vi "RT_Aerodynamic_Moment_due_to_Fins_Misalignment_2 (SubVI).vi"(5 "OUT_Interp":dbl[](array[numeric])=[0.0, 0.0, 0.0, 0.0, 0.0], 7 "input cluster 2":T3, 8 "Rotation":T1, 9 "i":i32, 10 "Vehicle Parameters":T2, 11 "Data":dbl[][](array[numeric])) -> (3 "MA_f":dbl[](array[numeric]))   [LabVIEW 2017]
uses:
  <vilib>/Analysis/baseanly.llb/Real A x B.vi
  <vilib>/Analysis/Matrix/Numeric/Conversions/Array To Matrix - RA2.vi
  <vilib>/Analysis/Matrix/Numeric/Conversions/Array To Matrix - RA.vi
  <vilib>/Analysis/Matrix/Numeric/Conversions/Matrix To Array - RM.vi
  <vilib>/Analysis/NI_AALBase.lvlib
  <vilib>/Analysis/Matrix/NI_Matrix.lvlib
panel:
  out "ma_f":dbl
  out "Cld":dbl
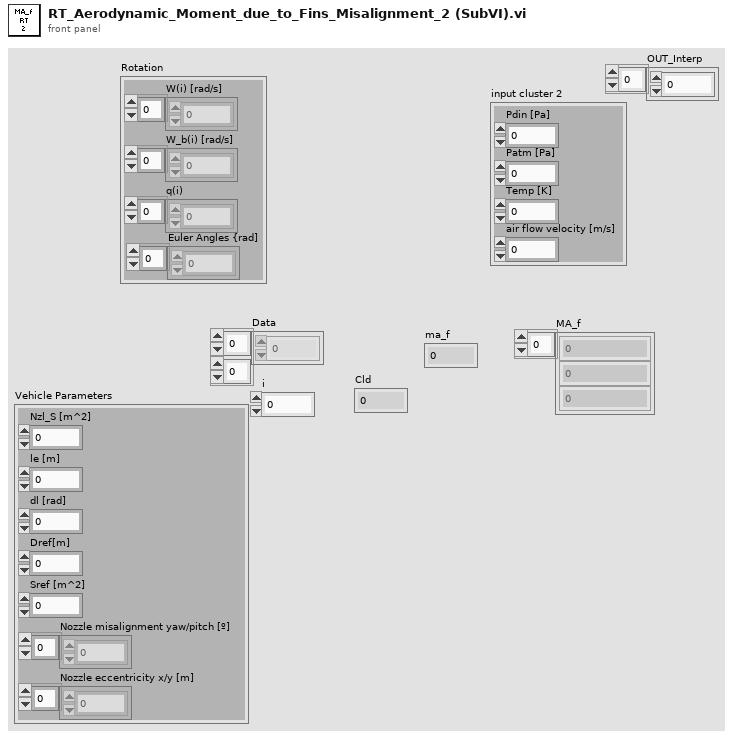
[diagram p1: front panel]
types:
  T1 = cluster{"W(i) [rad/s]":dbl[], "W_b(i) [rad/s]":dbl[], "q(i)":dbl[], "Euler Angles {rad]":dbl[]}
  T2 = cluster{"Nzl_S [m^2]":dbl, "le [m]":dbl, "dl [rad]":dbl, "Dref[m]":dbl, "Sref [m^2]":dbl, "Nozzle misalignment yaw/pitch [º]":dbl[], "Nozzle eccentricity x/y [m]":dbl[]}
  T3 = cluster{"Pdin [Pa]":dbl, "Patm [Pa]":dbl, "Temp [K]":dbl, "air flow velocity [m/s]":dbl}
  T4 = typedef "NI_Matrix.lvlib/RealMatrix.ctl" = dbl[][]
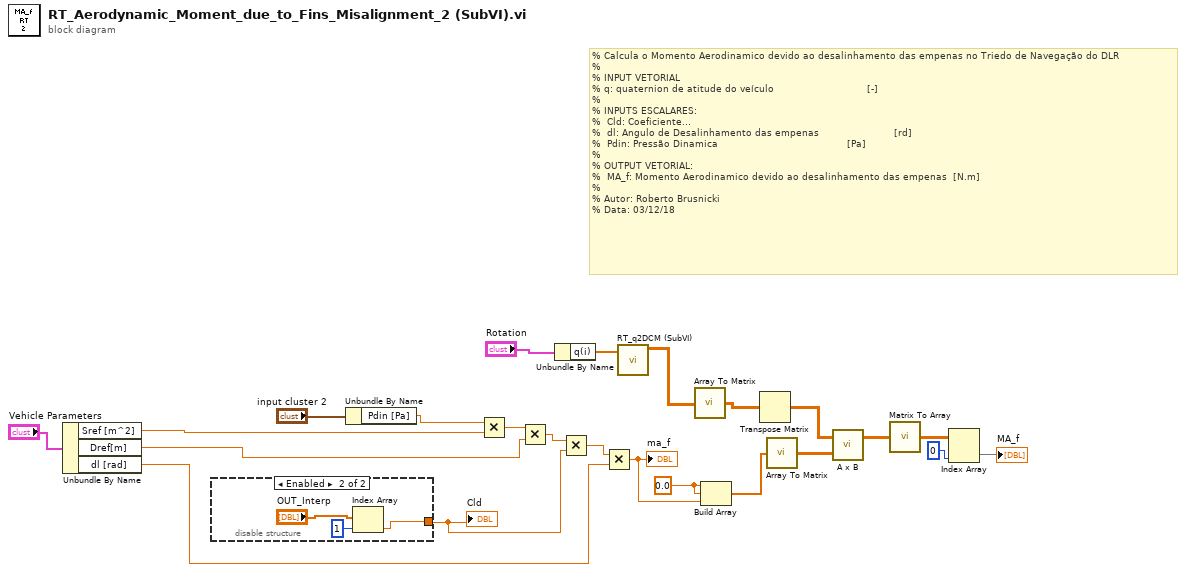
[diagram p0: block diagram]
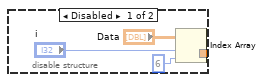
[diagram p2: hidden frame]
diagram:
  w16 = 0.0 ("element")
  # "% Calcula o Momento Aerodinamico devido ao desalinhamento das empenas no Triedo de Navegação do DLR\n%\n% INPUT VETORIAL\n% q: quaternion de atitude do veículo                               [-]\n%\n% INPUTS ESCALARES:\n%  Cld: Coeficiente...\n%  dl: Angulo de Desalinhamento das empenas                         [rd]\n%  Pdin: Pressão Dinamica                                           [Pa]\n%\n% OUTPUT VETORIAL:\n%  MA_f: Momento Aerodinamico devido ao desalinhamento das empenas  [N.m]\n%\n% Autor: Roberto Brusnicki\n% Data: 03/12/18"
  n1 = Unbundle By Name("Vehicle Parameters") -> ("Sref [m^2]"=w23:dbl, "Dref[m]"=w21:dbl, "dl [rad]"=w7:dbl)
  n2 = disable-structure shown="Enabled" {
    disable-tunnel: [w24 w29] -> w19
    frame Disabled {
      n3 = Index Array(array="Data", index (row)="i", index (col)=6 ("disabled index (col)")) -> (element=w24:dbl)
    }
    frame Enabled {
      n4 = Index Array(array="OUT_Interp", index=1) -> (element=w29:dbl)
    }
  }
  "Cld" <- w19
  n5 = Unbundle By Name("input cluster 2") -> ("Pdin [Pa]"=w6:dbl)
  n6 = Multiply(x=w6, y=w23) -> (x*y=w22:dbl)
  n7 = Multiply(x=w22, y=w21) -> (x*y=w20:dbl)
  n8 = Unbundle By Name("Rotation") -> ("q(i)"=w3:dbl[])
  n9 = Multiply(x=w20, y=w19) -> (x*y=w18:dbl)
  n10 = Multiply(x=w18, y=w7) -> (x*y=w17:dbl)
  "ma_f" <- w17
  n11 = call "RT_q2DCM (SubVI).vi"("Quaternion"=w3) -> ("DCM"=w2:dbl[][])  [unwired: 10 in]
  n12 = call-poly <vilib>:"Array To Matrix.vi"("Real 2D Array"=w2) -> ("Real Matrix"=w9:T4)
  n13 = Build Array(w16, w16, w17) -> (w10:dbl[])
  n14 = Transpose Matrix(1:w9) -> (0:w8:T4)
  n15 = call-poly <vilib>:"Array To Matrix.vi"("Real 1D Array"=w10) -> ("Real Matrix (Column Vector)"=w15:T4)
  n16 = call-poly <vilib>:"A x B.vi"("B"=w15, "A"=w8) -> ("A x B"=w13:T4)  [unwired: 1 out]
  n17 = call-poly <vilib>:"Matrix To Array.vi"("Real Matrix"=w13) -> ("Real 2D Array"=w14:dbl[][])
  n18 = Index Array(array=w14, index (col)=0 ("index (row)")) -> (element=→"MA_f":dbl[])  [unwired: 1 in]
